vi "Get Delay.vi"(8 "error in (no error)":errorcluster, 11 "Instrument.DelayLine in":refnum<class "Instrument.DelayLine.lvclass">) -> (0 "error out":errorcluster, 2 "Delay (ps)":dbl, 3 "Instrument.DelayLine out":refnum<class "Instrument.DelayLine.lvclass">, 4 "Finished?":bool)   [LabVIEW 2019, in "Instrument.DelayLine.lvclass"]
uses:
  Instrument.DelayLine.lvclass
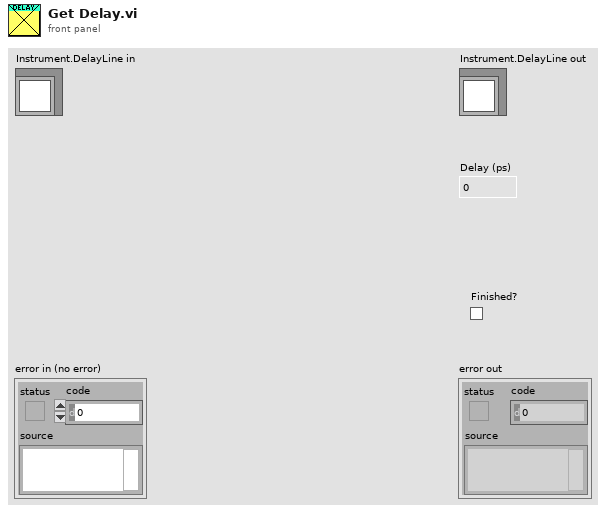
[diagram p1: front panel]
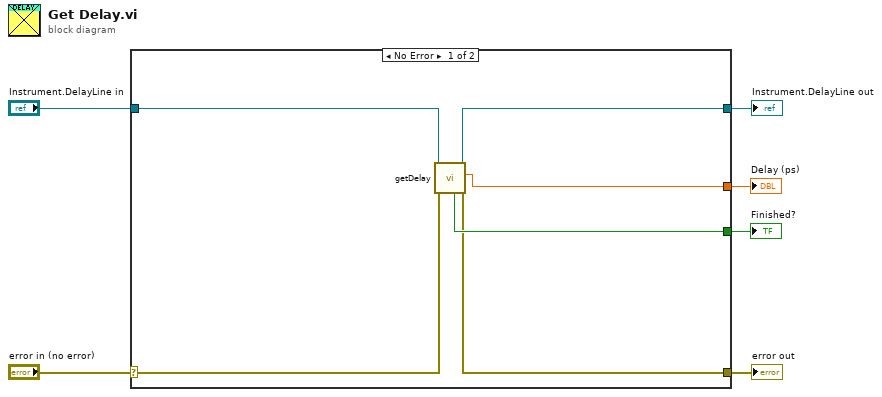
[diagram p0: block diagram]
diagram:
  n1 = case shown="No Error" "error in (no error)" {
    selector: "error in (no error)" -> [w8 w14]
    tunnel: [w7 w14] -> w5
    tunnel: [w12 w13] -> w3
    tunnel: "Instrument.DelayLine in" -> [w11 w13]
    tunnel: [w10 _] -> w2
    tunnel: [w9 _] -> w1
    frame No Error {
      n2 = call "getDelay.vi"("error in (no error)"=w8, "Instrument.DelayLine in"=w11) -> ("error out"=w7:errorcluster, "delay (ps)"=w10:dbl, "Instrument.DelayLine out"=w12:refnum<class "Instrument.DelayLine.lvclass">, "Finished?"=w9:bool)  [unwired: 6 in]
    }
    frame Error {
    }
  }
  "error out" <- w5
  "Instrument.DelayLine out" <- w3
  "Finished?" <- w1
  "Delay (ps)" <- w2
